vi "set filter (channel).vi"(5 "Use AND Logic? (False)":bool, 7 "Combine Existing (False)":bool, 8 "error in (no error)":errorcluster, 9 "Include Only Visible?":bool, 10 "Type":T1(ring), 11 "alias-tree in":refnum<class "alias-tree.lvclass">) -> (0 "error out":errorcluster, 3 "alias-tree out":refnum<class "alias-tree.lvclass">)   [LabVIEW 2017, in "vs-tree-utility.lvlib" / "alias-tree.lvclass"]
uses:
  alias-tree.lvclass
  NationalInstruments.VeriStand.SystemStorage
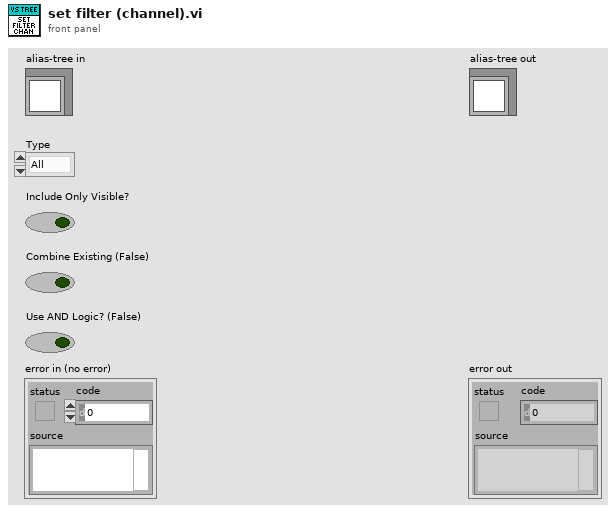
[diagram p1: front panel]
types:
  T1 = enum16{"All", "Readable", "Writeable", "Faultable", "Scalable"}
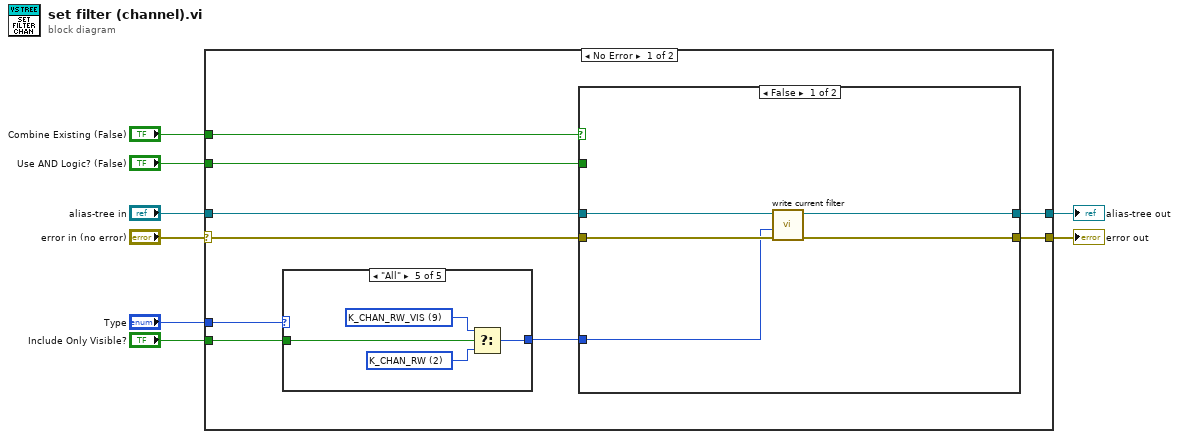
[diagram p0: block diagram]
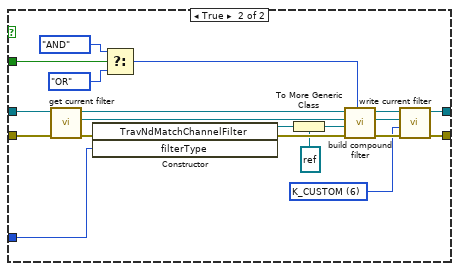
[diagram p2: hidden frame]
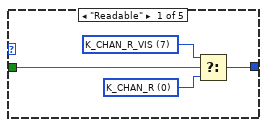
[diagram p3: hidden frame]
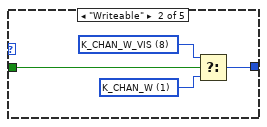
[diagram p4: hidden frame]
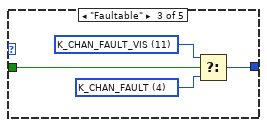
[diagram p5: hidden frame]
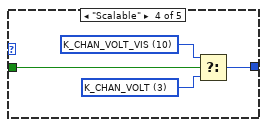
[diagram p6: hidden frame]
diagram:
  n1 = case shown="No Error" "error in (no error)" {
    selector: "error in (no error)" -> [w15 w64]
    tunnel: [w14 w64] -> w7
    tunnel: [w12 w63] -> w5
    tunnel: "alias-tree in" -> [w13 w63]
    tunnel: "Type" -> [w17 _]
    tunnel: "Include Only Visible?" -> [w16 _]
    tunnel: "Combine Existing (False)" -> [w10 _]
    tunnel: "Use AND Logic? (False)" -> [w9 _]
    frame No Error {
      n2 = case shown="\"All\"" w17 {
        tunnel: [w45 w49 w53 w57 w61] -> w11
        tunnel: w16 -> [w46 w50 w54 w58 w62]
        frame "Readable" {
          w43 = u8 0 items=["K_CHAN_R", "K_CHAN_W", "K_CHAN_RW", "K_CHAN_VOLT", "K_CHAN_FAULT", "K_ALL", "K_CUSTOM", "K_CHAN_R_VIS", "K_CHAN_W_VIS", "K_CHAN_RW_VIS", "K_CHAN_VOLT_VIS", "K_CHAN_FAULT_VIS", "K_WAVE", "K_WAVE_VIS", "K_WAVE_DBL", "K_WAVE_CDB", "K_WAVE_DBL_VIS", "K_WAVE_CDB_VIS"] ("filterType")
          w44 = u8 7 items=["K_CHAN_R", "K_CHAN_W", "K_CHAN_RW", "K_CHAN_VOLT", "K_CHAN_FAULT", "K_ALL", "K_CUSTOM", "K_CHAN_R_VIS", "K_CHAN_W_VIS", "K_CHAN_RW_VIS", "K_CHAN_VOLT_VIS", "K_CHAN_FAULT_VIS", "K_WAVE", "K_WAVE_VIS", "K_WAVE_DBL", "K_WAVE_CDB", "K_WAVE_DBL_VIS", "K_WAVE_CDB_VIS"] ("filterType")
          n3 = Select(t=w44, s=w46, f=w43) -> (s? t:f=w45:u8)
        }
        frame "Writeable" {
          w47 = u8 1 items=["K_CHAN_R", "K_CHAN_W", "K_CHAN_RW", "K_CHAN_VOLT", "K_CHAN_FAULT", "K_ALL", "K_CUSTOM", "K_CHAN_R_VIS", "K_CHAN_W_VIS", "K_CHAN_RW_VIS", "K_CHAN_VOLT_VIS", "K_CHAN_FAULT_VIS", "K_WAVE", "K_WAVE_VIS", "K_WAVE_DBL", "K_WAVE_CDB", "K_WAVE_DBL_VIS", "K_WAVE_CDB_VIS"] ("filterType")
          w48 = u8 8 items=["K_CHAN_R", "K_CHAN_W", "K_CHAN_RW", "K_CHAN_VOLT", "K_CHAN_FAULT", "K_ALL", "K_CUSTOM", "K_CHAN_R_VIS", "K_CHAN_W_VIS", "K_CHAN_RW_VIS", "K_CHAN_VOLT_VIS", "K_CHAN_FAULT_VIS", "K_WAVE", "K_WAVE_VIS", "K_WAVE_DBL", "K_WAVE_CDB", "K_WAVE_DBL_VIS", "K_WAVE_CDB_VIS"] ("filterType")
          n4 = Select(t=w48, s=w50, f=w47) -> (s? t:f=w49:u8)
        }
        frame "Faultable" {
          w51 = u8 4 items=["K_CHAN_R", "K_CHAN_W", "K_CHAN_RW", "K_CHAN_VOLT", "K_CHAN_FAULT", "K_ALL", "K_CUSTOM", "K_CHAN_R_VIS", "K_CHAN_W_VIS", "K_CHAN_RW_VIS", "K_CHAN_VOLT_VIS", "K_CHAN_FAULT_VIS", "K_WAVE", "K_WAVE_VIS", "K_WAVE_DBL", "K_WAVE_CDB", "K_WAVE_DBL_VIS", "K_WAVE_CDB_VIS"] ("filterType")
          w52 = u8 11 items=["K_CHAN_R", "K_CHAN_W", "K_CHAN_RW", "K_CHAN_VOLT", "K_CHAN_FAULT", "K_ALL", "K_CUSTOM", "K_CHAN_R_VIS", "K_CHAN_W_VIS", "K_CHAN_RW_VIS", "K_CHAN_VOLT_VIS", "K_CHAN_FAULT_VIS", "K_WAVE", "K_WAVE_VIS", "K_WAVE_DBL", "K_WAVE_CDB", "K_WAVE_DBL_VIS", "K_WAVE_CDB_VIS"] ("filterType")
          n5 = Select(t=w52, s=w54, f=w51) -> (s? t:f=w53:u8)
        }
        frame "Scalable" {
          w55 = u8 3 items=["K_CHAN_R", "K_CHAN_W", "K_CHAN_RW", "K_CHAN_VOLT", "K_CHAN_FAULT", "K_ALL", "K_CUSTOM", "K_CHAN_R_VIS", "K_CHAN_W_VIS", "K_CHAN_RW_VIS", "K_CHAN_VOLT_VIS", "K_CHAN_FAULT_VIS", "K_WAVE", "K_WAVE_VIS", "K_WAVE_DBL", "K_WAVE_CDB", "K_WAVE_DBL_VIS", "K_WAVE_CDB_VIS"] ("filterType")
          w56 = u8 10 items=["K_CHAN_R", "K_CHAN_W", "K_CHAN_RW", "K_CHAN_VOLT", "K_CHAN_FAULT", "K_ALL", "K_CUSTOM", "K_CHAN_R_VIS", "K_CHAN_W_VIS", "K_CHAN_RW_VIS", "K_CHAN_VOLT_VIS", "K_CHAN_FAULT_VIS", "K_WAVE", "K_WAVE_VIS", "K_WAVE_DBL", "K_WAVE_CDB", "K_WAVE_DBL_VIS", "K_WAVE_CDB_VIS"] ("filterType")
          n6 = Select(t=w56, s=w58, f=w55) -> (s? t:f=w57:u8)
        }
        frame "All" {
          w59 = u8 2 items=["K_CHAN_R", "K_CHAN_W", "K_CHAN_RW", "K_CHAN_VOLT", "K_CHAN_FAULT", "K_ALL", "K_CUSTOM", "K_CHAN_R_VIS", "K_CHAN_W_VIS", "K_CHAN_RW_VIS", "K_CHAN_VOLT_VIS", "K_CHAN_FAULT_VIS", "K_WAVE", "K_WAVE_VIS", "K_WAVE_DBL", "K_WAVE_CDB", "K_WAVE_DBL_VIS", "K_WAVE_CDB_VIS"] ("filterType")
          w60 = u8 9 items=["K_CHAN_R", "K_CHAN_W", "K_CHAN_RW", "K_CHAN_VOLT", "K_CHAN_FAULT", "K_ALL", "K_CUSTOM", "K_CHAN_R_VIS", "K_CHAN_W_VIS", "K_CHAN_RW_VIS", "K_CHAN_VOLT_VIS", "K_CHAN_FAULT_VIS", "K_WAVE", "K_WAVE_VIS", "K_WAVE_DBL", "K_WAVE_CDB", "K_WAVE_DBL_VIS", "K_WAVE_CDB_VIS"] ("filterType")
          n7 = Select(t=w60, s=w62, f=w59) -> (s? t:f=w61:u8)
        }
      }
      n8 = case shown="False" w10 {
        tunnel: w15 -> [w22 w38]
        tunnel: [w21 w33] -> w14
        tunnel: w13 -> [w20 w40]
        tunnel: [w19 w32] -> w12
        tunnel: w11 -> [w18 w29]
        tunnel: w9 -> [_ w41]
        frame False {
          n9 = call-dynamic "write current filter.vi"("error in (no error)"=w22, "filterType"=w18, "alias-tree in"=w20) -> ("error out"=w21:errorcluster, "alias-tree out"=w19:refnum<class "alias-tree.lvclass">)  [unwired: 7 in]
        }
        frame True {
          w31 = u8 6 items=["K_CHAN_R", "K_CHAN_W", "K_CHAN_RW", "K_CHAN_VOLT", "K_CHAN_FAULT", "K_ALL", "K_CUSTOM", "K_CHAN_R_VIS", "K_CHAN_W_VIS", "K_CHAN_RW_VIS", "K_CHAN_VOLT_VIS", "K_CHAN_FAULT_VIS", "K_WAVE", "K_WAVE_VIS", "K_WAVE_DBL", "K_WAVE_CDB", "K_WAVE_DBL_VIS", "K_WAVE_CDB_VIS"] ("filterType")
          n10 = call "get current filter.vi"("error in (no error)"=w38, "alias-tree in"=w40) -> ("error out"=w36:errorcluster, "display filter"=w27:refnum<k24>, "alias-tree out"=w37:refnum<class "alias-tree.lvclass">)  [unwired: 7 in]
          n11 = constructor class="TravNdMatchChannelFilter"(error in=w36, "filterType"=w29) -> (reference out=w28:refnum<k24>, error out=w30:errorcluster)  [unwired: 2 in, 2 out]
          n12 = Select(t=enum16{"AND", "OR"}."AND" ("Type (OR)"), s=w41, f=enum16{"AND", "OR"}."OR" ("Type (OR)")) -> (s? t:f=w23:enum16{"AND", "OR"})
          n13 = To More Generic Class(target class=refnum<k24> refnum, reference=w28) -> (generic class reference=w26:refnum<k24>)
          n14 = call-dynamic "build compound filter.vi"("Type (OR)"=w23, "error in (no error)"=w30, "Filter B"=w26, "Filter A"=w27, "alias-tree in"=w37) -> ("error out"=w35:errorcluster, "Compound Filter"=w24:refnum<k24>, "alias-tree out"=w34:refnum<class "alias-tree.lvclass">)  [unwired: 4 in]
          n15 = call-dynamic "write current filter.vi"("error in (no error)"=w35, "filterType"=w31, "Filter"=w24, "alias-tree in"=w34) -> ("error out"=w33:errorcluster, "alias-tree out"=w32:refnum<class "alias-tree.lvclass">)  [unwired: 6 in]
        }
      }
    }
    frame Error {
    }
  }
  "error out" <- w7
  "alias-tree out" <- w5
